vi "Configure Pulse.vi"(0 "VISA resource name":refnum<visa-resource-name>, 1 "Pulse Delay Increment (0 s)":dbl, 2 "Enable Pulse Output (F: Disable)":bool, 3 "Pulse Period (0.001 s)":dbl=0.001, 5 "Channel (1)":i32=1, 7 "Pulse Generator (1)":i32=1, 9 "Pulse Delay (0.0001 s)":dbl=0.0001, 11 "error in (no error)":errorcluster, 12 "Pulse Polarity (F: Disable)":bool, 13 "Pulse Width (0.0001 s)":dbl=0.0001) -> (4 "VISA resource name out":refnum<visa-resource-name>, 15 "error out":errorcluster)   [LabVIEW 2018, in "Keysight PNA Series.lvlib"]
doc: "Configures the 5 pulse generators in the PNA-X.\n\nNote:\nThis VI is only valid for PNA-X models."
uses:
  Keysight PNA Series.lvlib
panel:
  # "Note:\nThis VI is only valid for PNA-X models."
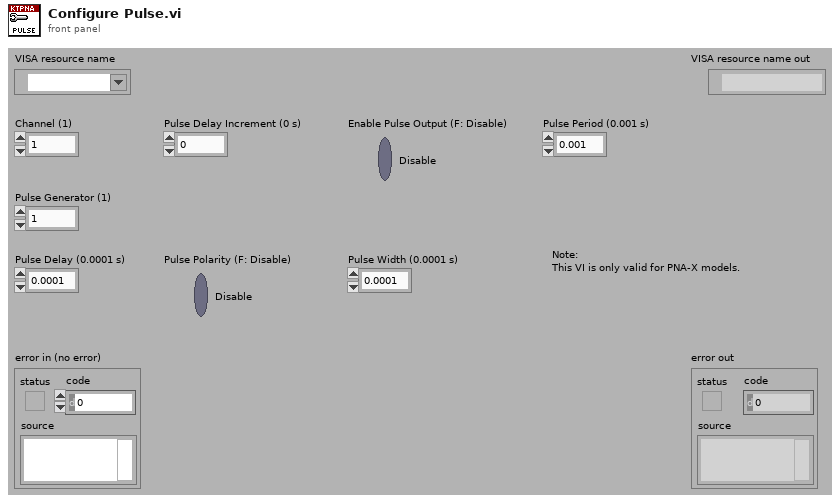
[diagram p1: front panel]
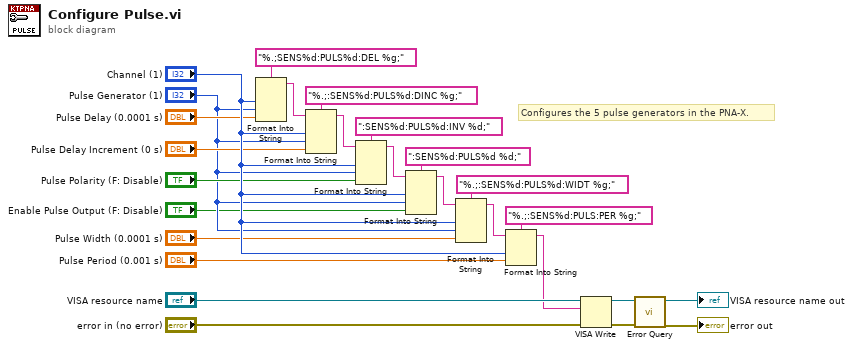
[diagram p0: block diagram]
diagram:
  # "Configures the 5 pulse generators in the PNA-X."
  n1 = Format Into String(format string="%.;SENS%d:PULS%d:DEL %g;", "Channel (1)", "Pulse Generator (1)", "Pulse Delay (0.0001 s)") -> (resulting string=w23:string)  [unwired: 2 in, 1 out]
  n2 = Format Into String(format string="%.;:SENS%d:PULS%d:DINC %g;", initial string=w23, "Channel (1)", "Pulse Generator (1)", "Pulse Delay Increment (0 s)") -> (resulting string=w20:string)  [unwired: 1 in, 1 out]
  n3 = Format Into String(format string=":SENS%d:PULS%d:INV %d;", initial string=w20, "Channel (1)", "Pulse Generator (1)", "Pulse Polarity (F: Disable)") -> (resulting string=w18:string)  [unwired: 1 in, 1 out]
  n4 = Format Into String(format string=":SENS%d:PULS%d %d;", initial string=w18, "Channel (1)", "Pulse Generator (1)", "Enable Pulse Output (F: Disable)") -> (resulting string=w16:string)  [unwired: 1 in, 1 out]
  n5 = Format Into String(format string="%.;:SENS%d:PULS%d:WIDT %g;", initial string=w16, "Channel (1)", "Pulse Generator (1)", "Pulse Width (0.0001 s)") -> (resulting string=w13:string)  [unwired: 1 in, 1 out]
  n6 = Format Into String(format string="%.;:SENS%d:PULS:PER %g;", initial string=w13, "Channel (1)", "Pulse Period (0.001 s)") -> (resulting string=w4:string)  [unwired: 1 in, 1 out]
  n7 = VISA Write(VISA resource name="VISA resource name", write buffer=w4, error in (no error)="error in (no error)") -> (VISA resource name out=w8:refnum<visa-resource-name>, error out=w7:errorcluster)  [unwired: 1 out]
  n8 = call "Error Query.vi"("error in (no error)"=w7, "VISA resource name"=w8) -> ("error out"=→"error out":errorcluster, "VISA resource name out"=→"VISA resource name out":refnum<visa-resource-name>)  [unwired: 6 in, 2 out]
